vi "Array.vi"() -> ()   [LabVIEW 2020]
panel:
  out "1D Horizontal New Array":dbl[](array[numeric])
  in  "New Element":dbl format="%#_13g"
  in  "index":i32
  in  "1D Horizontal Array":dbl[](array[numeric])
  out "1D Horizontal New Array":dbl[](array[numeric])
  in  "New Element":dbl format="%#_13g"
  in  "index":i32
  in  "1D Horizontal Array":dbl[](array[numeric])
  out "subarray column":dbl[](array[numeric])
  out "subarray row":dbl[](array[numeric])
  out "element 2":dbl
  in  "index column":i32
  in  "index row":i32
  in  "2D Array":dbl[][](array[numeric])
  out "element":dbl
  in  "index":i32
  in  "1D Horizontal Array":dbl[](array[numeric])
  out "2 arrays addition":dbl[](array[numeric])
  in  "1D Horizontal Array":dbl[](array[numeric])
  in  "1D Horizontal Array":dbl[](array[numeric])
  out "x+y":dbl[](array[numeric])
  out "appended appended array":dbl[][](array[numeric])
  out "appended array":dbl[][](array[numeric])
  in  "1D Horizontal Array":dbl[](array[numeric])
  in  "1D Horizontal Array":dbl[](array[numeric])
  in  "Size":i32
  in  "Element to be inserted":dbl format="%#_13g"
  out "initialized array":dbl[](array[numeric])
  out "2D Array Size":i32[](array[numeric])
  out "1D Vertical size":i32
  out "1D Horizontal size":i32
  out "2D Array Indicator 2":dbl[][](array[numeric])
  in  "2D Array":dbl[][](array[numeric])
  out "1D Vertical Array Indicator":dbl[](array[numeric])
  in  "1D Vertical Array Control":dbl[](array[numeric])
  in  "1D Horizontal Array":dbl[](array[numeric])
  # "Row             Column"
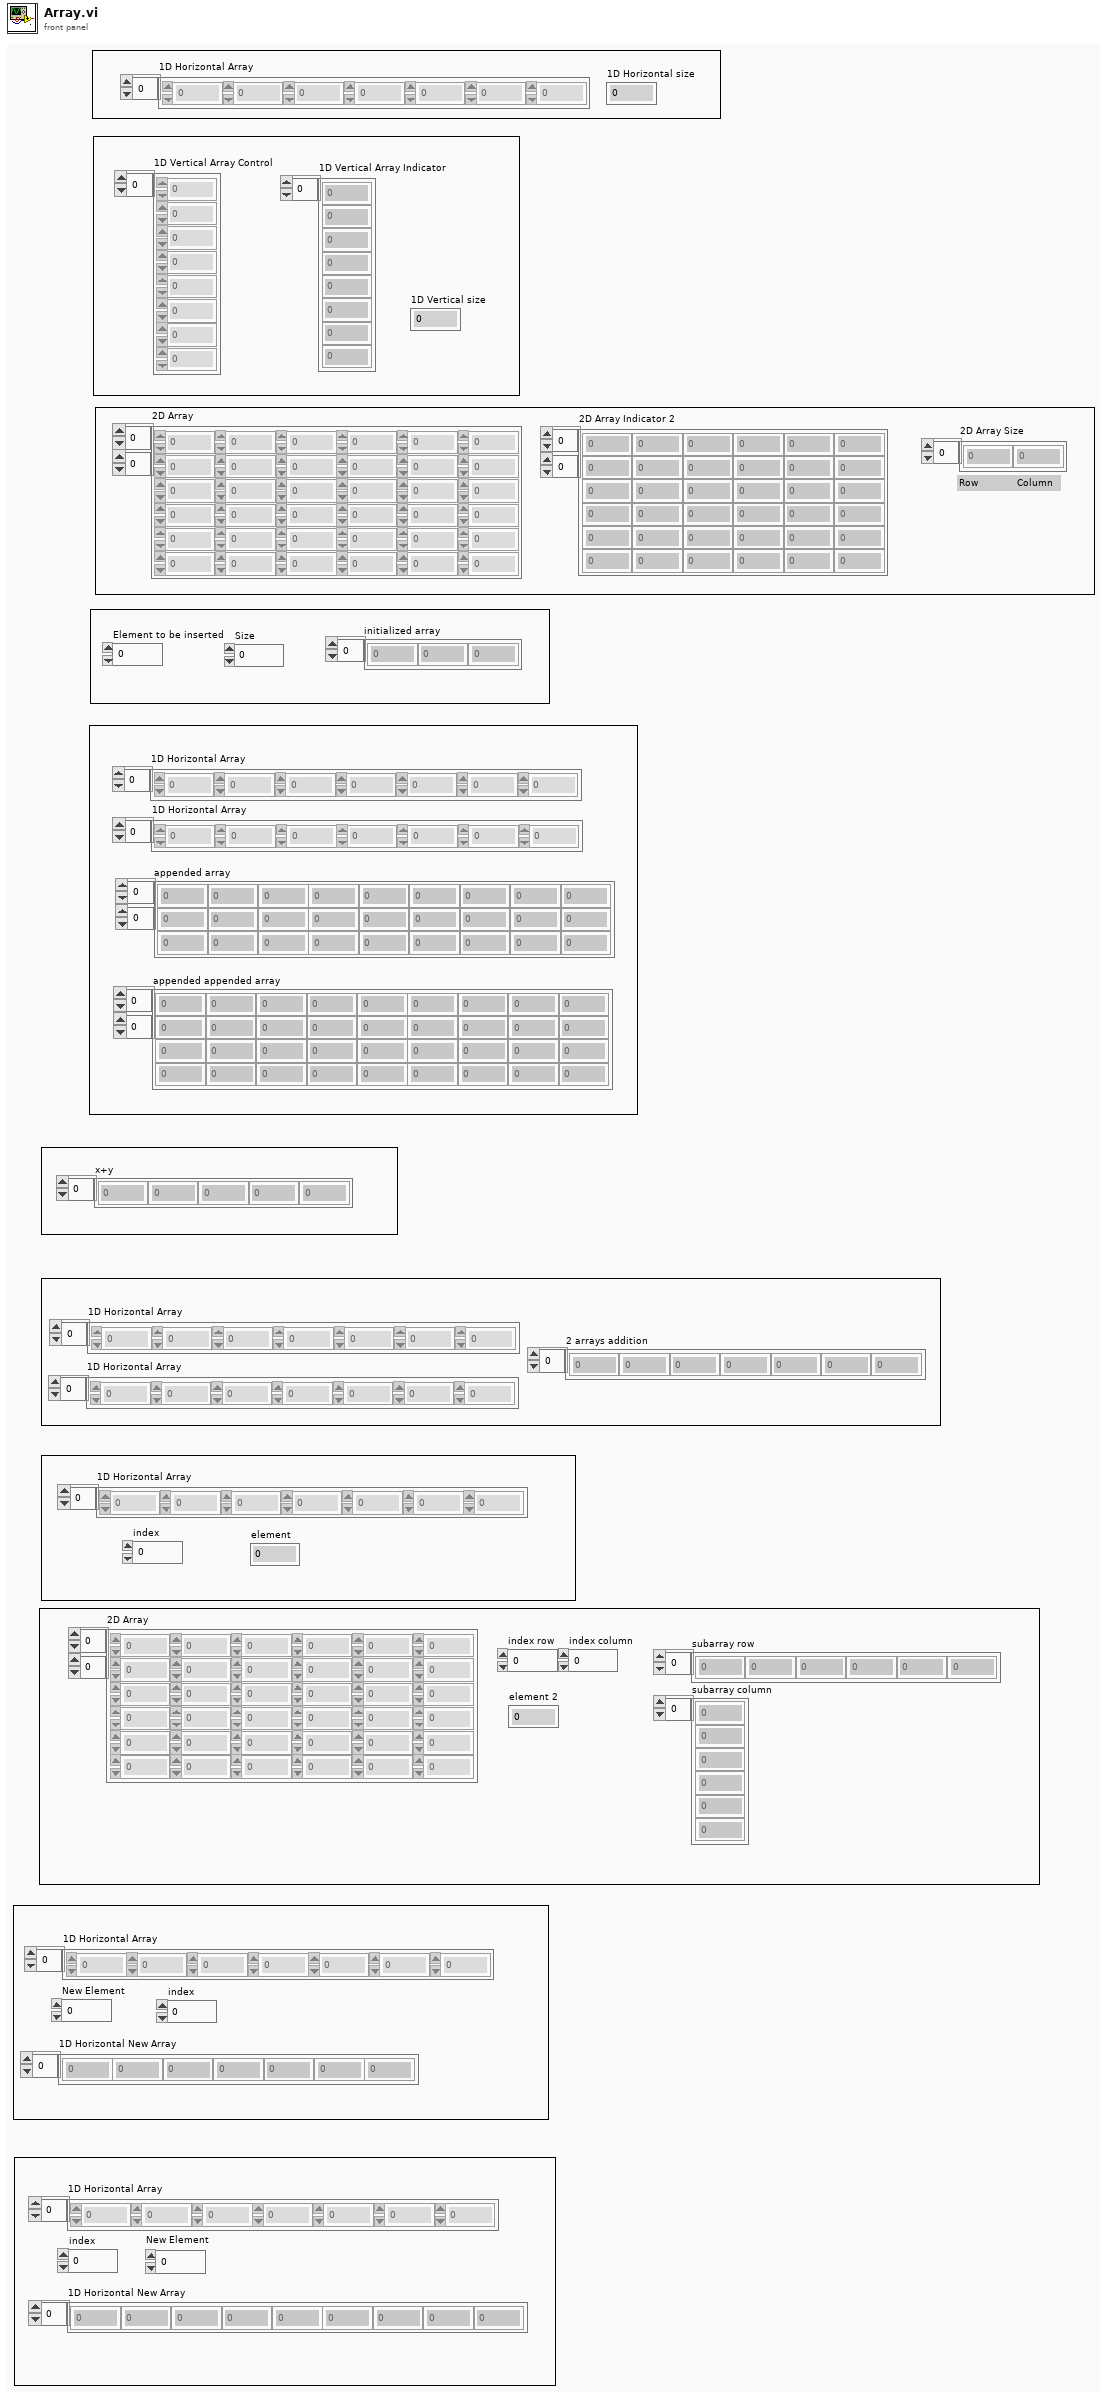
[diagram p1: front panel]
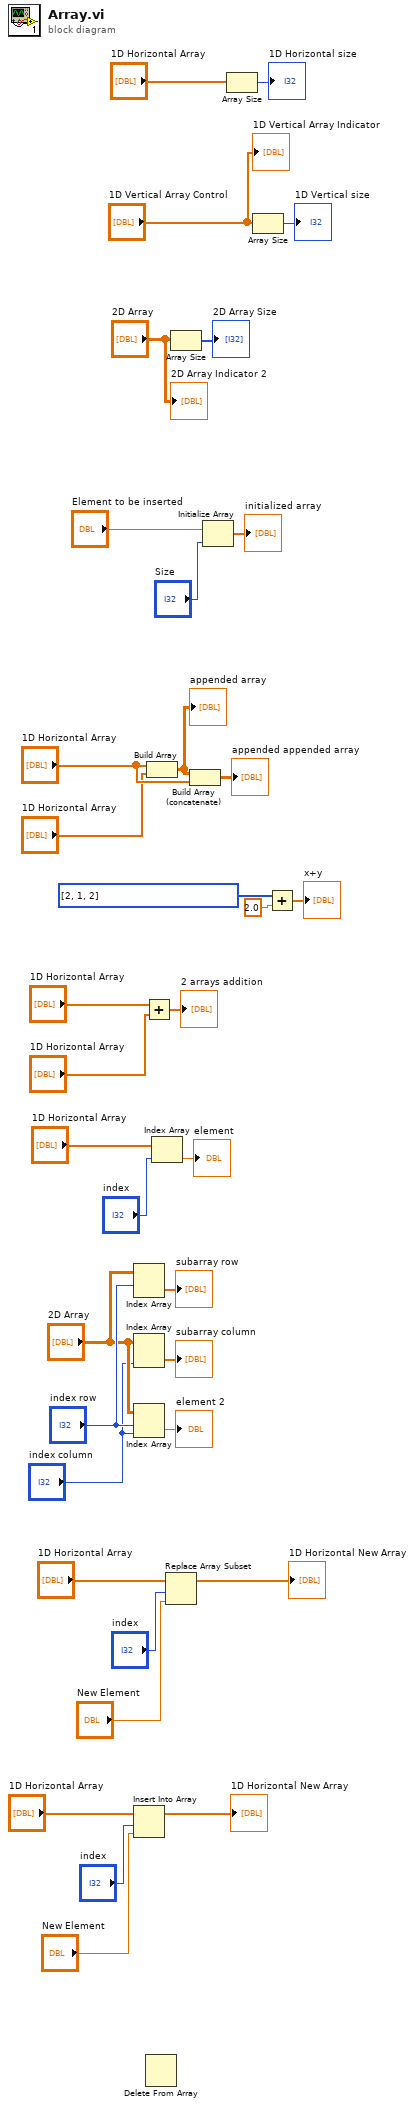
[diagram p0: block diagram]
diagram:
  n1 = Index Array(array="2D Array", index (row)="index row") -> (element=→"subarray row":dbl[])  [unwired: 1 in]
  n2 = Index Array(array="2D Array", index (col)="index column") -> (element=→"subarray column":dbl[])  [unwired: 1 in]
  n3 = Index Array(array="2D Array", index (row)="index row", index (col)="index column") -> (element=→"element 2":dbl)
  n4 = Insert Into Array "Insert Into Array"(array="1D Horizontal Array", index="index", new element="New Element") -> (→"1D Horizontal New Array":dbl[])
  n5 = Add(x="1D Horizontal Array", y="1D Horizontal Array") -> (x+y=→"2 arrays addition":dbl[])
  n6 = Delete From Array "Delete From Array"() -> ()  [unwired: 3 in, 2 out]
  n7 = Build Array("1D Horizontal Array", "1D Horizontal Array") -> (w24:dbl[][])
  "appended array" <- w24
  n8 = Index Array(array="1D Horizontal Array", index="index") -> (element=→"element":dbl)
  n9 = Replace Array Subset "Replace Array Subset"(array="1D Horizontal Array", new element="New Element", index="index") -> (→"1D Horizontal New Array":dbl[])
  n10 = Array Size(array="2D Array") -> (size(s)=→"2D Array Size":i32[])
  n11 = Build Array (concatenate)(w24, "1D Horizontal Array") -> (→"appended appended array":dbl[][])
  n12 = Initialize Array("Element to be inserted", "Size") -> (→"initialized array":dbl[])
  n13 = Array Size(array="1D Horizontal Array") -> (size(s)=→"1D Horizontal size":i32)
  n14 = Array Size(array="1D Vertical Array Control") -> (size(s)=→"1D Vertical size":i32)
  n15 = Add(x=i32[] [2, 1, 2], y=2.0) -> (x+y=→"x+y":dbl[])
  "1D Vertical Array Indicator" <- "1D Vertical Array Control"
  "2D Array Indicator 2" <- "2D Array"
